vi "GetClass - Window Info.vi"(5 "error in (no error)":errorcluster) -> (13 "Window Info":T1(array[cluster]), 19 "error out":errorcluster)   [LabVIEW 2020, in "SPWB.lvclass"]
uses:
  SPWB.lvclass
  API/GSwFormDSP_class/GSwFormDSP.lvclass
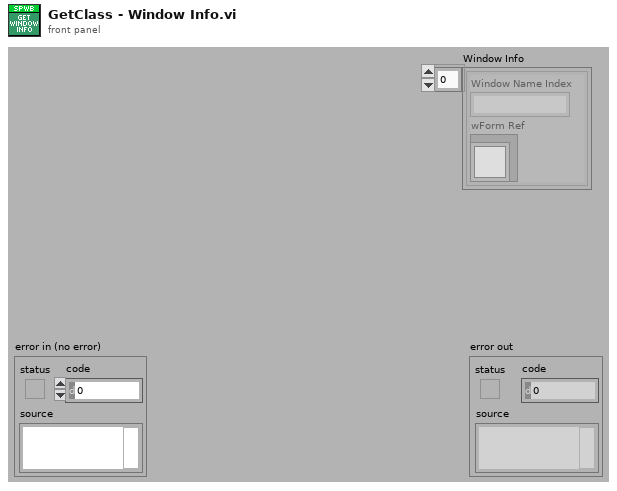
[diagram p1: front panel]
types:
  T1 = cluster{"Window Name Index":string, "wForm Ref":refnum<class "GSwFormDSP.lvclass">}[]
  T2 = typedef "SPWB.lvclass/ClassAttributes.ctl" = cluster{"Window Info":cluster{"Window Name Index":string, "wForm Ref":refnum<class "GSwFormDSP.lvclass">}[]}
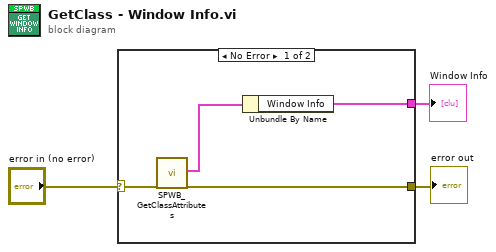
[diagram p0: block diagram]
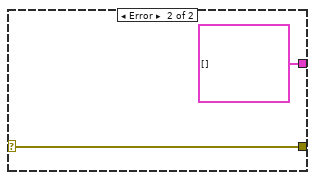
[diagram p2: hidden frame]
diagram:
  n1 = case shown="No Error" "error in (no error)" {
    selector: "error in (no error)" -> [w7 w9]
    tunnel: [w6 w9] -> w2
    tunnel: [w4 T1 [] ("Window Info")] -> w1
    frame No Error {
      n2 = call "SPWB_GetClassAttributes.vi"("error in (no error)"=w7) -> ("class attributes"=w5:T2, "error out"=w6:errorcluster)  [unwired: 15 in, 2 out]
      n3 = Unbundle By Name(w5) -> ("Window Info"=w4:T1)
    }
    frame Error {
    }
  }
  "error out" <- w2
  "Window Info" <- w1
